vi "Read CAN Xnet.vi"(4 "error in":errorcluster, 5 "XNET Communications Properties":T1 {"CAN I/O Mode" items=["CAN", "CAN FD", "CAN FD + BRS"]}, 6 "Tlg Data Array":T3 {"CAN frame In"."FlexRay"."cycle count" max=63 step=1; "CAN frame In"."payload" format="%x"; "CAN frame In"."identifier / slot" format="%x"; "FlexRay Channel" items=["A", "B", "A+B"]}, 7 "NewData In":bool) -> (0 "error out":errorcluster, 1 "XNET Communications Properties Out":T1 {"CAN I/O Mode" items=["CAN", "CAN FD", "CAN FD + BRS"]}, 2 "Tlg Data Array out":T3 {"CAN frame In"."FlexRay"."cycle count" max=63 step=1; "CAN frame In"."payload" format="%x"; "CAN frame In"."identifier / slot" format="%x"; "FlexRay Channel" items=["A", "B", "A+B"]}, 3 "NewData":bool)   [LabVIEW 2014, in "CAN Bus Monitor Engine.lvlib"]
uses:
  CAN Bus Monitor Engine.lvlib
  Controls/Analyze Array.ctl
  Controls/FlexRay Channel.ctl
  Controls/XNET BM Frame.ctl
  Controls/XNET Communication Properties.ctl
  Controls/CAN IO Mode.ctl
  <vilib>/xnet/xnet.llb/XNET Read (Frame Raw).vi
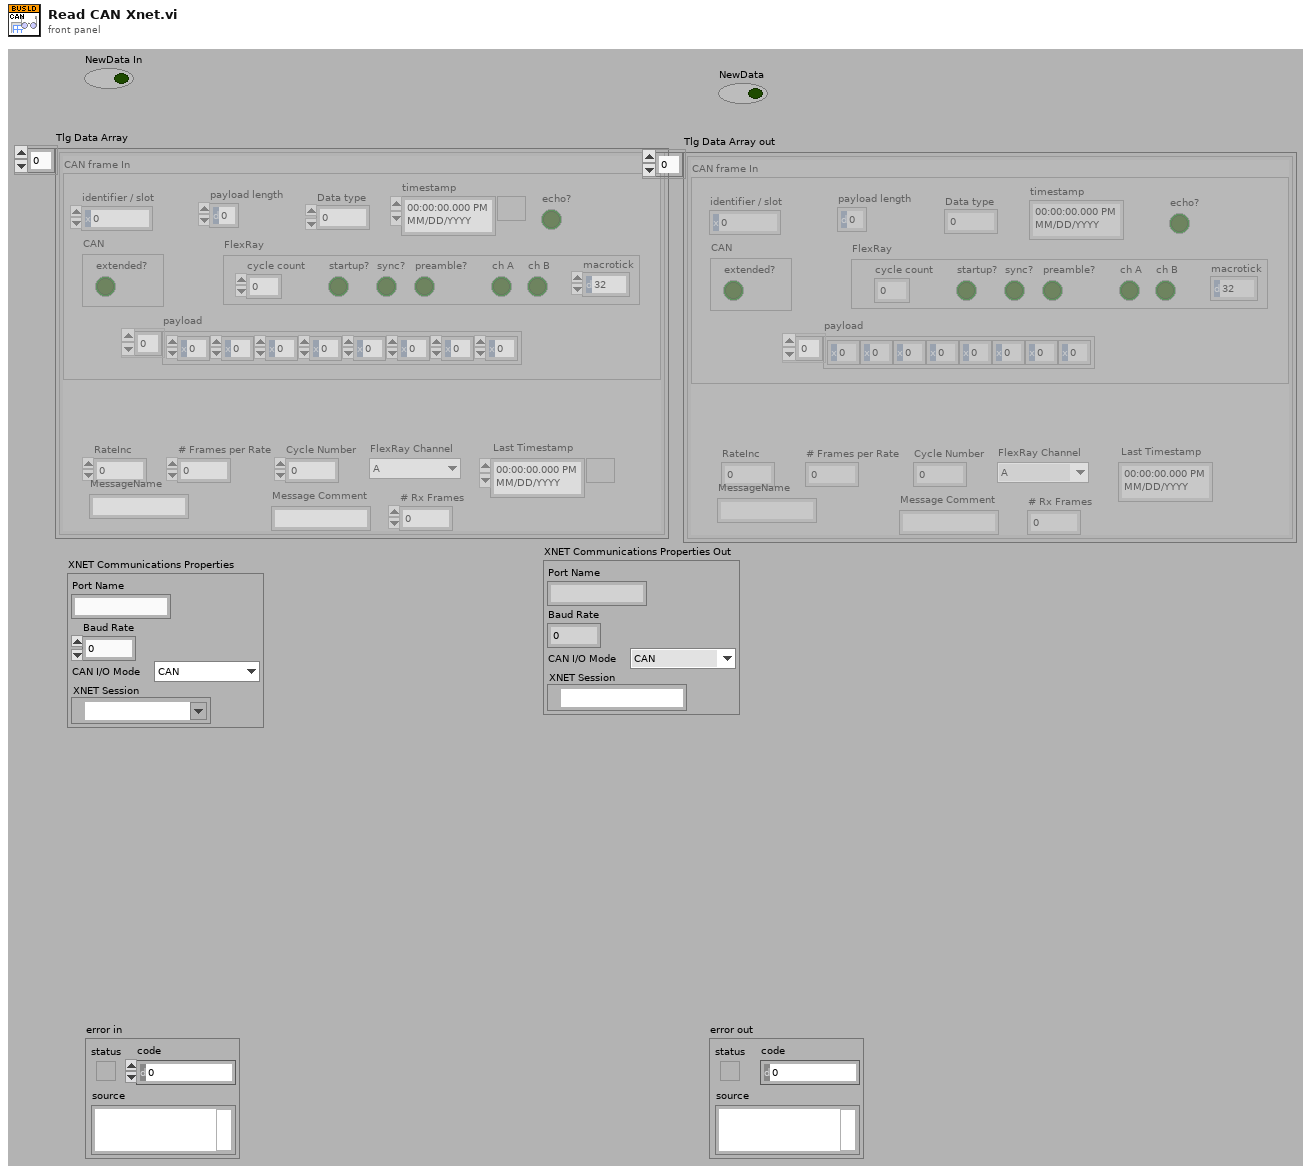
[diagram p1: front panel]
types:
  T1 = typedef "CAN Bus Monitor Engine.lvlib/XNET Communication Properties.ctl" = cluster{"Port Name":string, "Baud Rate":u32, "CAN I/O Mode":T2, "XNET Session":refnum<k21>}
  T2 = typedef "CAN Bus Monitor Engine.lvlib/CAN IO Mode.ctl" = u32
  T3 = typedef "CAN Bus Monitor Engine.lvlib/Analyze Array.ctl" = cluster{"# Rx Frames":u32, "Last Timestamp":timestamp, "RateInc":dbl, "# Frames per Rate":u32, "MessageName":string, "Cycle Number":u32, "FlexRay Channel":T4, "Message Comment":string, "CAN frame In":T5}[]
  T4 = typedef "CAN Bus Monitor Engine.lvlib/FlexRay Channel.ctl" = u16
  T5 = typedef "CAN Bus Monitor Engine.lvlib/XNET BM Frame.ctl" = cluster{"timestamp":timestamp, "payload":u8[], "identifier / slot":u32, "Data type":u8, "payload length":u8, "CAN":cluster{"extended?":bool}, "FlexRay":cluster{"cycle count":u8, "startup?":bool, "sync?":bool, "preamble?":bool, "ch A":bool, "ch B":bool, "macrotick":u16}, "echo?":bool}
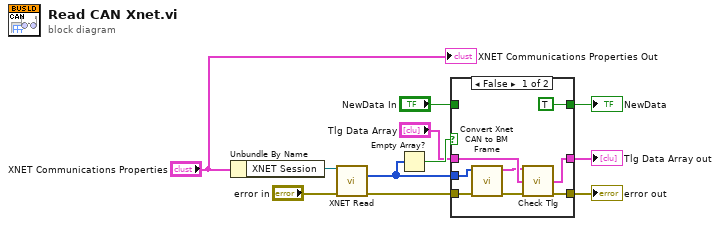
[diagram p0: block diagram]
diagram:
  n1 = Unbundle By Name("XNET Communications Properties") -> ("XNET Session"=w9:refnum<k21>)
  n2 = call-poly <vilib>:"XNET Read.vi"("session in"=w9, "error in (no error)"="error in") -> ("data"=w4:u8[], "error out"=w6:errorcluster)  [unwired: 11 in, 1 out]
  n3 = Empty Array?(array=w4) -> (empty?=w5:bool)
  n4 = case shown="False" w5 {
    tunnel: [TRUE ("NewData") w22] -> w2
    tunnel: [w12 w21] -> w11
    tunnel: "Tlg Data Array" -> [w18 w20]
    tunnel: [w17 w20] -> w10
    tunnel: w6 -> [w14 w21]
    tunnel: "NewData In" -> [_ w22]
    tunnel: w4 -> [w15 _]
    frame False {
      n5 = call "Convert Xnet CAN to BM Frame.vi"("error in"=w14, "CAN Raw Data"=w15) -> ("error out"=w13:errorcluster, "BM Frame Out"=w16:T5[])  [unwired: 8 in]
      n6 = call "Check Tlg.vi"("Data Read In"=w16, "Tlg Data Array"=w18, "Error In"=w13) -> ("Tlg Data Array out"=w17:T3, "Error out"=w12:errorcluster)  [unwired: 10 in, 1 out]
    }
    frame True {
    }
  }
  "NewData" <- w2
  "error out" <- w11
  "Tlg Data Array out" <- w10
  "XNET Communications Properties Out" <- "XNET Communications Properties"
